vi "Configure PLL.vi"(7 "instance":i32, 8 "error in":errorcluster, 10 "config":T1, 11 "lia host in":refnum<class "LIA Host Interface.lvclass">) -> (0 "error out":errorcluster, 3 "lia host out":refnum<class "LIA Host Interface.lvclass">)   [LabVIEW 2017, in "LIA Host Interface.lvclass"]
uses:
  LIA Host Interface.lvclass
  host/Public/pll settings.ctl
  host/Lock-In Amplifier Example Host.lvlib
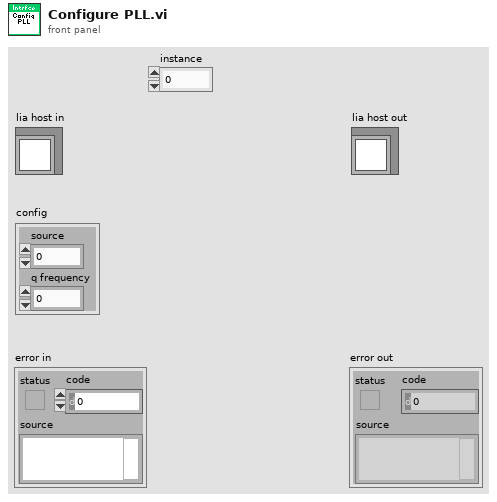
[diagram p1: front panel]
types:
  T1 = typedef "Lock-In Amplifier Example Host.lvlib/pll settings.ctl" = cluster{"source":i32, "q frequency":dbl}
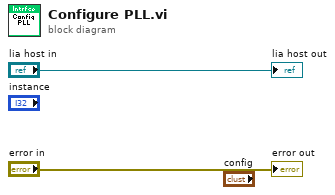
[diagram p0: block diagram]
diagram:
  "error out" <- "error in"
  "lia host out" <- "lia host in"
